vi "BMcalculate_v1_3 (slide_fix).vi"() -> ()   [LabVIEW 2014]
uses:
  <vilib>/Analysis/coordinate.llb/2D Cartesian Coordinate Rotation (Array).vi
  <vilib>/Analysis/baseanly.llb/Mean (DBL).vi
  <vilib>/Utility/file.llb/Read From Spreadsheet File (string).vi
  <vilib>/Utility/file.llb/Write To Spreadsheet File (DBL).vi
  <vilib>/Analysis/NI_AALBase.lvlib
  <vilib>/Analysis/NI_AALPro.lvlib
panel:
  in  "(T=X , F=Y)":bool=TRUE
  in  "Filter window size":i32=100
  out "Array":dbl[](array[numeric])
  out "created path 2":path
  out "created path":path
  in  "Save Time-trace":bool
  in  "nm/pixel":dbl=72.5 format="%#_13g"
  in  "Folder path":path
  in  "?":bool
  in  "~":dbl=1.15 format="%#_13g"
  in  "x/y for all":dbl=0.85 format="%#_13g"
  out "filename":string
  in  "Filter mode":T1(ring)=enum."Median_slide window"
  in  "Save to vertical data ?":bool
  in  "?":enum32{"slide by slide", "delay"}(tab)=enum."delay"
  in  "?":bool
  in  "seconds to wait":u32
  in  "?":dbl=7.963 format="%#_13g"
  in  "?":dbl=48.61 format="%#_13g"
  in  "Save BM":bool
  in  "?":bool=TRUE
  in  "Save X-Y plot":bool
  in  "less than":dbl=0.2 format="%#_13g"
  in  "?":bool
  in  "?":bool
  in  "?":bool=TRUE
  in  "?":T2(tab)
  out "Filenames":string[](array[string])
  out "useful AOIs":i32[](array[numeric])
  out "# of AOI":i32[](array[numeric])
  out "% of useful AOIs":dbl
  out "tt # of AOIs":i32
  out "# of Frames":dbl[](array[numeric])
  out "tt # 0f useful AOIs":i32
  out "?":T3(graph)
  out "size(s)":i32
  out "X-Y plot":cluster{dbl[], dbl[]}(graph)
  out "Xstd":dbl
  out "ystd":dbl[](array[numeric])
  out "X":dbl format="%0.2f"
  out "Y":dbl format="%0.2f"
  out "?":T3(graph)
  out "tt # of useful AOIs":i32
  out "xstd":dbl[](array[numeric])
  out "# of AOI":i32
  out "y 2":dbl[](array[numeric])
  out "# of frames":dbl
  out "all y position (pixel)":dbl[][](array[numeric])
  out "all x position (pixel)":dbl[][](array[numeric])
  out "y":dbl[](array[numeric])
  out "x":dbl[](array[numeric])
  out "y":dbl[](array[numeric])
  out "x":dbl[](array[numeric])
  out "number":dbl[][](array[numeric])
  out "all rows":string[][](array[string])
  out "Useful aoi number":string[][](array[string])
  in  "Tab Control":enum32{"Time trace"}(tab)
  out "Time trace":T4(graph)
  in  "Highlight":dbl=30.0
  in  "±":dbl=30.0
  out "aoi":string
  # "Critiria"
  # "±"
  # "nm"
  # "for ssDNA strande exchange \n                    23.776±6.613 nm"
  # "for D-loop  (90+4)\n                    48.61±7.963 nm"
  # "for D-loop  (150+4)\n                    49.57±8.56 nm"
  # "nm"
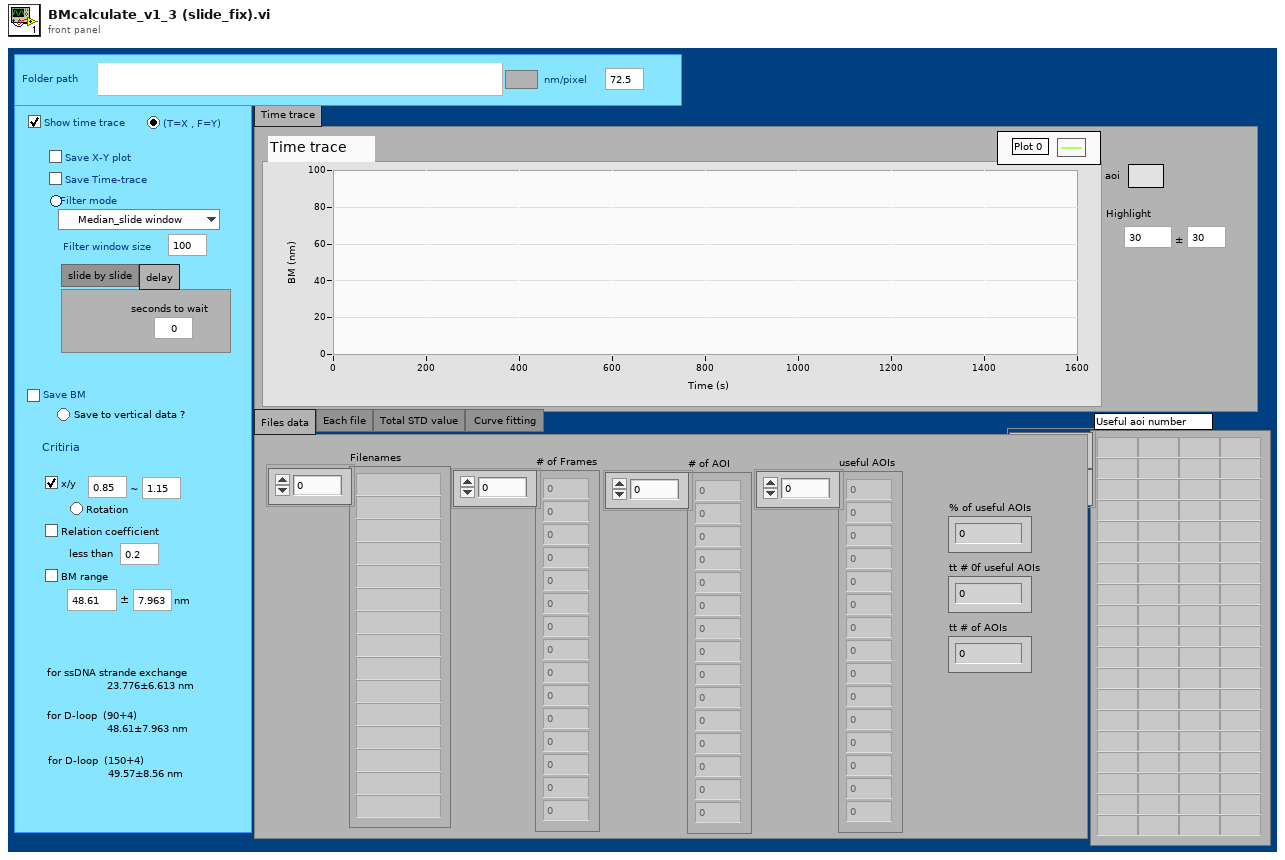
[diagram p1: front panel]
types:
  T1 = enum16{"Median_fix window", "Average_fix window", "Median_slide window", "Average_slide window"}
  T2 = enum32{"Files data", "Each file", "Total STD value", "Curve fitting "}
  T3 = cluster{"X Values":dbl[], "Histogram: h(x)":i32[]}
  T4 = cluster{"Filtered X":dbl[], "Filtered X":dbl[]}[]
  T5 = cluster{"all y position (pixel)":dbl[], "all x position (pixel)":dbl[]}
  T6 = cluster{"all x position (pixel)":dbl[], "all y position (pixel)":dbl[]}
  T7 = typedef "imagedata.ctl" = cluster{"image type":i32, "image depth":i32, "image":u8[], "mask":u8[], "colors":u32[], "Rectangle":cluster{"left":i16, "top":i16, "right":i16, "bottom":i16}}
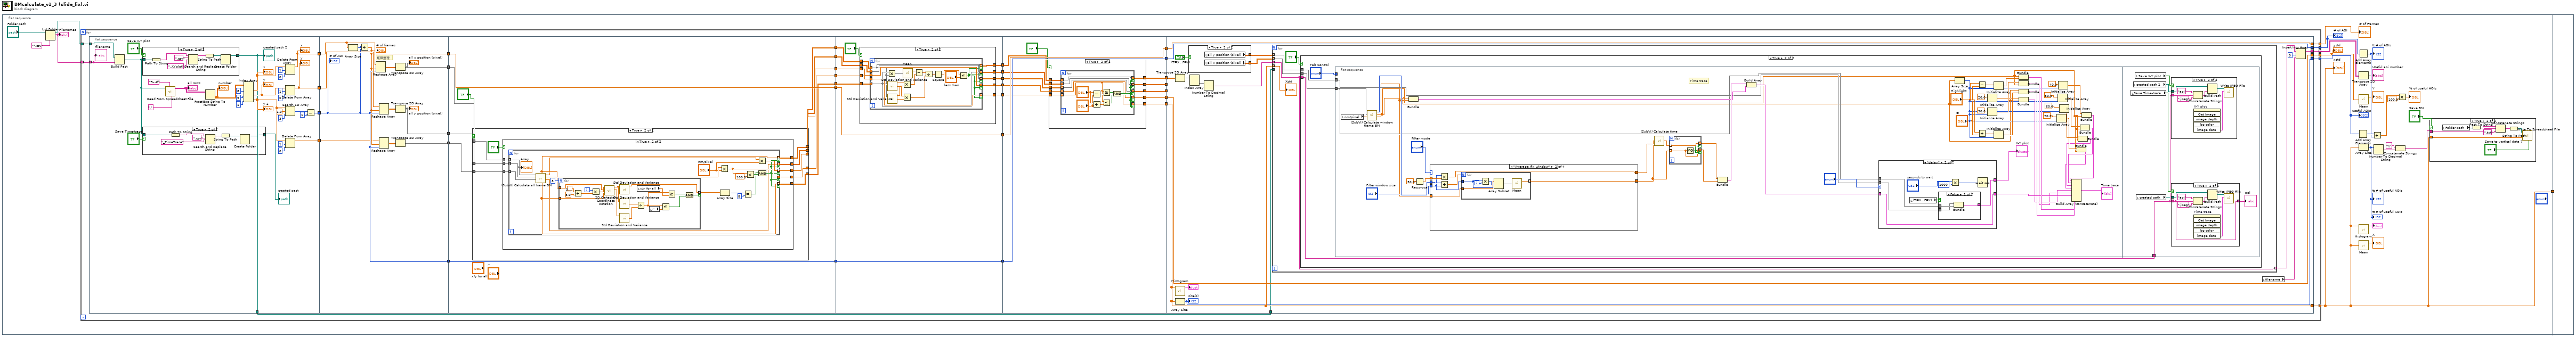
[diagram p0: block diagram]
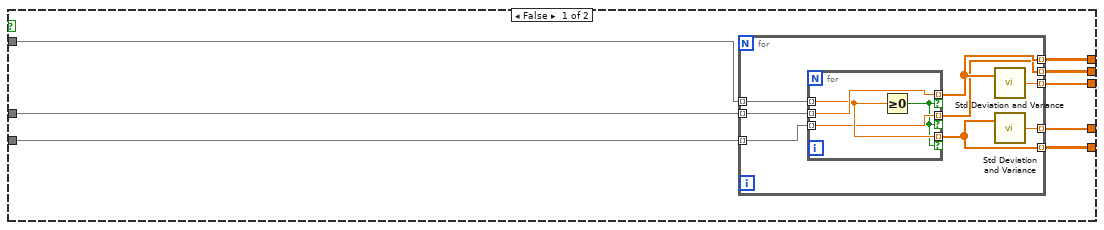
[diagram p5: hidden frame]
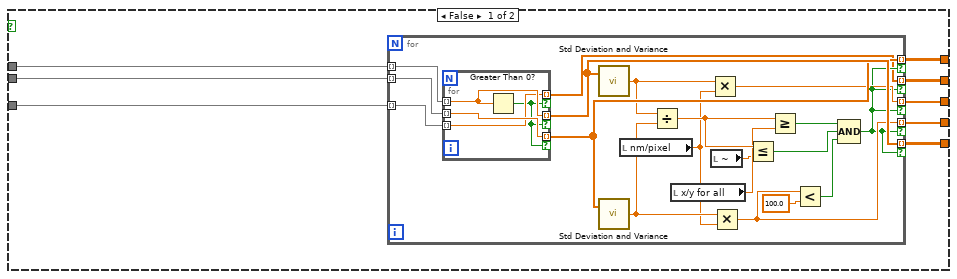
[diagram p6: hidden frame]
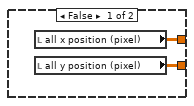
[diagram p9: hidden frame]
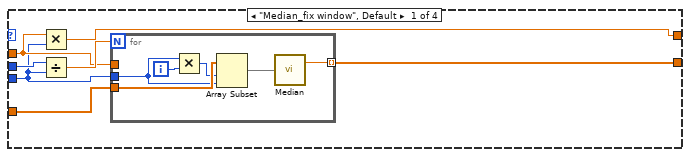
[diagram p11: hidden frame]
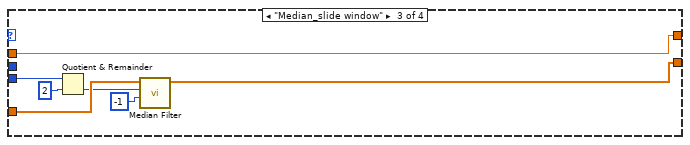
[diagram p12: hidden frame]
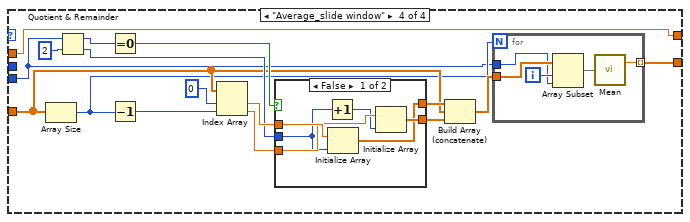
[diagram p13: hidden frame]
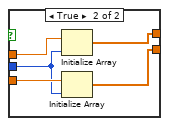
[diagram p14: hidden frame]
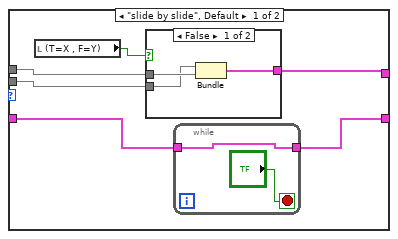
[diagram p15: hidden frame]
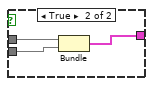
[diagram p16: hidden frame]
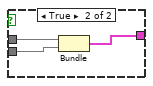
[diagram p17: hidden frame]
diagram:
  n1 = flat-sequence {
    tunnel: [w2] -> w1
    tunnel: w1 -> [_]
    frame #0 {
      n2 = List Folder(path="Folder path", pattern="*.csv") -> (path out=w24:path, filenames=w23:string[])  [unwired: 2 in, 2 out]
      "Filenames" <- w23
      n3 = for {
        tunnel: w24 -> [w37]
        tunnel: w23 -> [w72] mode=indexing
        tunnel: [w71] -> w2 mode=concatenating
        tunnel: [w70] -> w21 mode=indexing
        tunnel: [w69] -> w20 mode=indexing
        tunnel: [w68] -> w12 mode=concatenating
        tunnel: [w67] -> w13 mode=indexing
        tunnel: [w34] -> w4 mode=indexing
        n4 = flat-sequence {
          tunnel: [w92] -> w66
          tunnel: [w91] -> w65
          tunnel: [w85] -> w64
          tunnel: w37 -> [w80]
          tunnel: w72 -> [w76]
          tunnel: [w81] -> w41
          tunnel: [w79] -> w35
          tunnel: w66 -> [w128]
          tunnel: w65 -> [w127]
          tunnel: w64 -> [w126]
          tunnel: [w125] -> w63
          tunnel: [w126] -> w62
          tunnel: [w121] -> w61
          tunnel: [w120] -> w60
          tunnel: w41 -> [w124]
          tunnel: [w122] -> w40
          tunnel: w63 -> [w142]
          tunnel: w62 -> [w141]
          tunnel: w61 -> [w140]
          tunnel: w60 -> [w139]
          tunnel: [w141] -> w53
          tunnel: [w142] -> w51
          tunnel: [w137] -> w49
          tunnel: [w136] -> w47
          tunnel: [w135] -> w45
          tunnel: [w134] -> w43
          tunnel: w40 -> [w132]
          tunnel: [w133] -> w39
          tunnel: w53 -> [w260]
          tunnel: [w260] -> w52
          tunnel: w51 -> [w259]
          tunnel: [w259] -> w50
          tunnel: w49 -> [w255]
          tunnel: [w250] -> w48
          tunnel: w47 -> [w258]
          tunnel: [w253] -> w46
          tunnel: w45 -> [w257]
          tunnel: [w252] -> w44
          tunnel: w43 -> [w256]
          tunnel: [w251] -> w42
          tunnel: w39 -> [w249]
          tunnel: [w248] -> w38
          tunnel: w52 -> [w306]
          tunnel: w50 -> [w305]
          tunnel: w48 -> [w300]
          tunnel: [w306] -> w59
          tunnel: [w305] -> w58
          tunnel: [w299] -> w57
          tunnel: [w303] -> w56
          tunnel: w46 -> [w304]
          tunnel: [w301] -> w55
          tunnel: w44 -> [w302]
          tunnel: [w294] -> w54
          tunnel: w42 -> [w295]
          tunnel: w38 -> [w297]
          tunnel: [w296] -> w36
          tunnel: [w351] -> w68
          tunnel: [w352] -> w67
          tunnel: [w353] -> w69
          tunnel: [w349] -> w70
          tunnel: [w343] -> w71
          tunnel: w59 -> [w353]
          tunnel: w58 -> [w352]
          tunnel: w57 -> [w351]
          tunnel: w56 -> [_]
          tunnel: w55 -> [_]
          tunnel: w54 -> [w343]
          tunnel: w36 -> [w348]
          tunnel: w35 -> [w344]
          tunnel: [w339] -> w34
          frame #0 {
            n5 = Build Path(base path=w80, name or relative path=w76) -> (appended path=w74:path)
            n6 = case shown="True" "Save X-Y plot" {
              tunnel: w74 -> [w112 w119]
              tunnel: [w112 w113] -> w79
              frame False {
              }
              frame True {
                n7 = Path To String(path=w119) -> (string=w118:string)
                n8 = Search and Replace String(input string=w118, search string=".csv", replace string="_XYplot" ("replace string (\"\")")) -> (result string=w115:string)  [unwired: 5 in, 3 out]
                n9 = String To Path(string=w115) -> (path=w114:path)
                n10 = Create Folder(path (use dialog)=w114) -> (created path=w113:path)  [unwired: 2 in, 2 out]
              }
            }
            "created path 2" <- w79
            n11 = case shown="True" "Save Time-trace" {
              tunnel: w74 -> [w104 w111]
              tunnel: [w104 w105] -> w73
              frame False {
              }
              frame True {
                n12 = Path To String(path=w111) -> (string=w110:string)
                n13 = Search and Replace String(input string=w110, search string=".csv", replace string="_TimeTrace" ("replace string (\"\")")) -> (result string=w107:string)  [unwired: 5 in, 3 out]
                n14 = String To Path(string=w107) -> (path=w106:path)
                n15 = Create Folder(path (use dialog)=w106) -> (created path=w105:path)  [unwired: 2 in, 2 out]
              }
            }
            "created path" <- w73
            n16 = call-poly <vilib>:"Read From Spreadsheet File.vi"("delimiter (\\t)"="," ("delimiter (\\t)"), "format (%s)"="%.4f" ("format (%.3f)"), "file path (dialog if empty)"=w74) -> ("all rows"=w102:string[][])  [unwired: 4 in, 4 out]
            "all rows" <- w102
            n17 = Fract/Exp String To Number(string=w102) -> (number=w101:dbl[][])  [unwired: 3 in, 1 out]
            "number" <- w101
            n18 = Index Array(array=w101, index (col) #1=8 ("disabled index (col)"), index (col) #2=9 ("index (col)"), index (col) #3=1 ("index (col)")) -> (element #1=w93:dbl[], element #2=w94:dbl[], element #3=w82:dbl[])  [unwired: 3 in]
            "x" <- w93
            "y" <- w94
            "y 2" <- w82
            n19 = Delete From Array(array=w93, length=1, index=0) -> (array with subset deleted=w92:dbl[])  [unwired: 1 out]
            "x" <- w92
            n20 = Delete From Array(array=w94, length=1, index=0) -> (array with subset deleted=w91:dbl[])  [unwired: 1 out]
            "y" <- w91
            n21 = Search 1D Array(1D array=w82, element=1.0, start index (0)=3) -> (index of element=w87:i32)
            n22 = Delete From Array(array=w82, length=1, index=0) -> (array with subset deleted=w81:dbl[])  [unwired: 1 out]
            n23 = Subtract(x=w87, y=1) -> (x-y=w85:i32)
            "filename" <- w76
          }
          frame #1 {
            # "矩陣整理"
            n24 = Array Size(array=w128) -> (size(s)=w129:i32)
            n25 = Divide(x=w129, y=w126) -> (x/y=w125:dbl)
            "# of frames" <- w125
            n26 = Reshape Array(w128, w125, w126) -> (w130:dbl[][])
            n27 = Reshape Array(w127, w125, w126) -> (w131:dbl[][])
            n28 = Reshape Array(w124, w125, w126) -> (w123:dbl[][])
            n29 = Transpose 2D Array(2D array=w130) -> (transposed array=w121:dbl[][])
            "all x position (pixel)" <- w121
            n30 = Transpose 2D Array(2D array=w131) -> (transposed array=w120:dbl[][])
            "all y position (pixel)" <- w120
            n31 = Transpose 2D Array(2D array=w123) -> (transposed array=w122:dbl[][])
            "# of AOI" <- w126
          }
          frame #2 {
            n32 = case shown="True" "?" {
              tunnel: [w148 w171] -> w136
              tunnel: [w147 w170] -> w135
              tunnel: w140 -> [w150 w169]
              tunnel: w139 -> [w149 w168]
              tunnel: [w146 w167] -> w134
              tunnel: [w145 w166] -> w137
              tunnel: w132 -> [w144 w164]
              tunnel: [w143 w163] -> w133
              frame False {
                n33 = for {
                  tunnel: w150 -> [w158] mode=indexing
                  tunnel: w149 -> [w157] mode=indexing
                  tunnel: [w156] -> w148 mode=indexing
                  tunnel: [w155] -> w147 mode=indexing
                  tunnel: [w154] -> w146 mode=indexing
                  tunnel: [w153] -> w145 mode=indexing
                  tunnel: w144 -> [w152] mode=indexing
                  tunnel: [w151] -> w143 mode=indexing
                  n34 = for {
                    tunnel: w158 -> [w161] mode=indexing
                    tunnel: w157 -> [w162] mode=indexing
                    tunnel: [w161] -> w156 mode=indexing if=w159
                    tunnel: [w162] -> w155 mode=indexing if=w159
                    tunnel: w152 -> [w160] mode=indexing
                    tunnel: [w160] -> w151 mode=indexing if=w159
                    n35 = Greater Or Equal To 0?(x=w161) -> (x >= 0?=w159:bool)
                  }
                  n36 = call <vilib>:"Std Deviation and Variance.vi"("X"=w155) -> ("standard deviation"=w153:dbl)  [unwired: 1 in, 2 out]
                  n37 = call <vilib>:"Std Deviation and Variance.vi"("X"=w156) -> ("standard deviation"=w154:dbl)  [unwired: 1 in, 2 out]
                }
              }
              frame True {
                n38 = case shown="True" "?" {
                  tunnel: w168 -> [w178 w210]
                  tunnel: w169 -> [w179 w209]
                  tunnel: [w177 w208] -> w171
                  tunnel: [w176 w207] -> w170
                  tunnel: [w175 w206] -> w167
                  tunnel: [w174 w205] -> w166
                  tunnel: w164 -> [w173 w204]
                  tunnel: [w172 w203] -> w163
                  frame False {
                    n39 = for {
                      tunnel: w179 -> [w198] mode=indexing
                      tunnel: w178 -> [w197] mode=indexing
                      tunnel: [w196] -> w177 mode=indexing if=w183
                      tunnel: [w195] -> w176 mode=indexing if=w183
                      tunnel: [w184] -> w175 mode=indexing if=w183
                      tunnel: [w187] -> w174 mode=indexing if=w183
                      tunnel: [w181] -> w172 mode=indexing if=w183
                      tunnel: w173 -> [w182] mode=indexing
                      n40 = for {
                        tunnel: w198 -> [w201] mode=indexing
                        tunnel: w197 -> [w202] mode=indexing
                        tunnel: [w201] -> w196 mode=indexing if=w199
                        tunnel: [w202] -> w195 mode=indexing if=w199
                        tunnel: w182 -> [w200] mode=indexing
                        tunnel: [w200] -> w181 mode=indexing if=w199
                        n41 = Greater Than 0?(x=w201) -> (x > 0?=w199:bool)
                      }
                      n42 = call <vilib>:"Std Deviation and Variance.vi"("X"=w196) -> ("standard deviation"=w188:dbl)  [unwired: 1 in, 2 out]
                      n43 = call <vilib>:"Std Deviation and Variance.vi"("X"=w195) -> ("standard deviation"=w189:dbl)  [unwired: 1 in, 2 out]
                      n44 = local read "nm/pixel"() -> (w180:dbl)
                      n45 = Divide(x=w188, y=w189) -> (x/y=w194:dbl)
                      n46 = local read "x/y for all"() -> (w193:dbl)
                      n47 = Multiply(x=w188, y=w180) -> (x*y=w187:dbl)
                      n48 = local read "~"() -> (w192:dbl)
                      n49 = Multiply(x=w189, y=w180) -> (x*y=w184:dbl)
                      n50 = Less Or Equal?(x=w194, y=w192) -> (x <= y?=w190:bool)
                      n51 = Greater Or Equal?(x=w194, y=w193) -> (x >= y?=w191:bool)
                      n52 = Less?(x=w184, y=100.0) -> (x < y?=w185:bool)
                      n53 = Compound Arithmetic op=AND(w191, w190, w185) -> (w183:bool)
                    }
                  }
                  frame True {
                    n54 = for {
                      tunnel: w209 -> [w229] mode=indexing
                      tunnel: w210 -> [w228] mode=indexing
                      tunnel: [w214] -> w206 mode=indexing if=w213
                      tunnel: [w221] -> w207 mode=indexing if=w213
                      tunnel: [w222] -> w208 mode=indexing if=w213
                      tunnel: [w219] -> w205 mode=indexing if=w213
                      tunnel: [w212] -> w203 mode=indexing if=w213
                      tunnel: w204 -> [w211] mode=indexing
                      n55 = call "(SubVI) Calculate all frame BM.vi"("AOI label"=w211, "y position (pixel)"=w228, "x position (pixel)"=w229) -> ("Array out"=w212:dbl[], "standard deviation 2"=w223:dbl, "standard deviation"=w220:dbl, "Array 4"=w222:dbl[], "Array 3"=w221:dbl[])  [unwired: 4 in]
                      n56 = for {
                        N: 8 -> [_]
                        tunnel: w222 -> [w242]
                        tunnel: w221 -> [w241]
                        tunnel: [w233] -> w224 mode=indexing if=w232
                        i -> [w243]
                        n57 = Divide(x=3.141592653589793, y=8.0) -> (x/y=w246:dbl)
                        n58 = Multiply(x=w243, y=w246) -> (x*y=w244:dbl)
                        n59 = call-poly <vilib>:"2D Cartesian Coordinate Rotation.vi"("theta"=w244, "Y"=w241, "X"=w242) -> ("Y Out"=w234:dbl[], "X Out"=w235:dbl[])  [unwired: 6 in, 1 out]
                        n60 = call <vilib>:"Std Deviation and Variance.vi"("X"=w235) -> ("mean"=w233:dbl)  [unwired: 1 in, 2 out]
                        n61 = call <vilib>:"Std Deviation and Variance.vi"("X"=w235) -> ("standard deviation"=w240:dbl)  [unwired: 1 in, 2 out]
                        n62 = call <vilib>:"Std Deviation and Variance.vi"("X"=w234) -> ("standard deviation"=w239:dbl)  [unwired: 1 in, 2 out]
                        n63 = Divide(x=w240, y=w239) -> (x/y=w238:dbl)
                        n64 = local read "x/y for all"() -> (w231:dbl)
                        n65 = local read "~"() -> (w230:dbl)
                        n66 = Less Or Equal?(x=w238, y=w230) -> (x <= y?=w236:bool)
                        n67 = Greater Or Equal?(x=w238, y=w231) -> (x >= y?=w237:bool)
                        n68 = Compound Arithmetic op=AND(w237, w236) -> (w232:bool)
                      }
                      n69 = Multiply(x=w223, y="nm/pixel") -> (x*y=w214:dbl)
                      n70 = Array Size(array=w224) -> (size(s)=w226:i32)
                      n71 = Equal?(x=w226, y=8) -> (x = y?=w215:bool)
                      n72 = Less?(x=w214, y=100.0) -> (x < y?=w216:bool)
                      n73 = Multiply(x=w220, y="nm/pixel") -> (x*y=w219:dbl)
                      n74 = Compound Arithmetic op=AND(w215, w216) -> (w213:bool)
                      "Array" <- w229
                    }
                  }
                }
              }
            }
          }
          frame #3 {
            n75 = case shown="True" "?" {
              tunnel: w258 -> [w265 w275]
              tunnel: w257 -> [w264 w274]
              tunnel: w256 -> [w263 w271]
              tunnel: w255 -> [w262 w269]
              tunnel: [w265 w273] -> w253
              tunnel: [w264 w272] -> w252
              tunnel: [w263 w270] -> w251
              tunnel: [w262 w268] -> w250
              tunnel: w249 -> [w261 w267]
              tunnel: [w261 w266] -> w248
              frame False {
              }
              frame True {
                n76 = for {
                  tunnel: w275 -> [w281] mode=indexing
                  tunnel: w274 -> [w280] mode=indexing
                  tunnel: [w281] -> w273 mode=indexing if=w276
                  tunnel: [w280] -> w272 mode=indexing if=w276
                  tunnel: [w288] -> w270 mode=indexing if=w276
                  tunnel: w271 -> [w288] mode=indexing
                  tunnel: w269 -> [w287] mode=indexing
                  tunnel: [w287] -> w268 mode=indexing if=w276
                  tunnel: [w277] -> w266 mode=indexing if=w276
                  tunnel: w267 -> [w277] mode=indexing
                  n77 = Multiply(x=w281, y=w280) -> (x*y=w279:dbl[])
                  n78 = call <vilib>:"Std Deviation and Variance.vi"("X"=w281) -> ("mean"=w284:dbl, "standard deviation"=w286:dbl)  [unwired: 1 in, 1 out]
                  n79 = call <vilib>:"Std Deviation and Variance.vi"("X"=w280) -> ("mean"=w283:dbl, "standard deviation"=w285:dbl)  [unwired: 1 in, 1 out]
                  n80 = Multiply(x=w284, y=w283) -> (x*y=w282:dbl)
                  n81 = Multiply(x=w286, y=w285) -> (x*y=w289:dbl)
                  n82 = call-poly <vilib>:"Mean.vi"("X"=w279) -> ("mean"=w278:dbl)  [unwired: 1 out]
                  n83 = Subtract(x=w278, y=w282) -> (x-y=w290:dbl)
                  n84 = Divide(x=w290, y=w289) -> (x/y=w291:dbl)
                  n85 = Square(x=w291) -> (x^2=w292:dbl)
                  n86 = Less Or Equal?(x=w292, y="less than") -> (x <= y?=w276:bool)
                }
              }
            }
          }
          frame #4 {
            n87 = case shown="True" "?" {
              tunnel: [w312 w322] -> w303
              tunnel: w304 -> [w312 w323]
              tunnel: w302 -> [w311 w321]
              tunnel: [w311 w320] -> w301
              tunnel: w295 -> [w310 w319]
              tunnel: [w310 w318] -> w294
              tunnel: w300 -> [w309 w317]
              tunnel: [w309 w316] -> w299
              tunnel: w297 -> [w308 w315]
              tunnel: [w307 w314] -> w296
              frame False {
                n88 = for {
                  tunnel: w308 -> [w313] mode=indexing
                  tunnel: [w313] -> w307 mode=indexing
                }
              }
              frame True {
                n89 = for {
                  tunnel: [w335] -> w322 mode=indexing if=w330
                  tunnel: w323 -> [w335] mode=indexing
                  tunnel: [w334] -> w320 mode=indexing if=w330
                  tunnel: w321 -> [w334] mode=indexing
                  tunnel: [w324] -> w318 mode=indexing if=w330
                  tunnel: w319 -> [w324] mode=indexing
                  tunnel: w317 -> [w329] mode=indexing
                  tunnel: [w329] -> w316 mode=indexing if=w330
                  tunnel: [w331] -> w314 mode=indexing if=w330
                  tunnel: w315 -> [w331] mode=indexing
                  n90 = Subtract(x="?", y="?") -> (x-y=w326:dbl)
                  n91 = Add(x="?", y="?") -> (x+y=w325:dbl)
                  n92 = Greater Or Equal?(x=w324, y=w326) -> (x >= y?=w333:bool)
                  n93 = Less Or Equal?(x=w324, y=w325) -> (x <= y?=w332:bool)
                  n94 = Compound Arithmetic op=AND(w333, w332) -> (w330:bool)
                }
              }
            }
          }
          frame #5 {
            n95 = Transpose 2D Array(2D array=w348) -> (transposed array=w347:dbl[][])
            n96 = call <vilib>:"Histogram.vi"("X"=w343) -> ("Histogram Graph"=→"?":T3)  [unwired: 7 in, 3 out]
            n97 = Array Size(array=w343) -> (size(s)=w349:i32)
            "size(s)" <- w349
            n98 = case shown="True" "(T=X , F=Y)" {
              tunnel: [w355 w357] -> w337
              tunnel: [w354 w356] -> w336
              frame False {
                n99 = local read "all x position (pixel)"() -> (w354:dbl[][])
                n100 = local read "all y position (pixel)"() -> (w355:dbl[][])
              }
              frame True {
                n101 = local read "all y position (pixel)"() -> (w356:dbl[][])
                n102 = local read "all x position (pixel)"() -> (w357:dbl[][])
              }
            }
            n103 = Index Array(array=w347) -> (element=w346:dbl[])  [unwired: 2 in]
            n104 = Number To Decimal String(number=w346) -> (decimal integer string=w345:string[])  [unwired: 1 in]
            n105 = for {
              tunnel: w337 -> [w361] mode=indexing
              tunnel: w336 -> [w362] mode=indexing
              tunnel: w345 -> [w358] mode=indexing
              tunnel: w344 -> [_]
              tunnel: w343 -> [w359] mode=indexing
              tunnel: [w358] -> w340 mode=indexing
              n106 = case shown="True" "?" {
                tunnel: w362 -> [_ w366]
                tunnel: w361 -> [_ w365]
                tunnel: w358 -> [_ w364]
                frame False {
                }
                frame True {
                  n107 = flat-sequence {
                    tunnel: w366 -> [w406]
                    tunnel: w365 -> [w405]
                    tunnel: "Tab Control" -> [_]
                    tunnel: w364 -> [w516]
                    frame #0 {
                      # "Time trace"
                      n108 = local read "nm/pixel"() -> (w393:dbl)
                      n109 = call "(SubVI) Calculate window frame BM.vi"("nm/pixel"=w393, "all x position (pixel)"=w405) -> ("BM"=w388:dbl[], "sec"=w371:dbl[], "frame"=w411:i32)  [unwired: 3 in]
                      n110 = Bundle("sec"=w371, "BM"=w388) -> (w410:cluster{"sec":dbl[], "BM":dbl[]})  [unwired: 1 in]
                      n111 = Reciprocal(x=30.0) -> (1/x=w390:dbl)
                      n112 = case shown="\"Average_fix window\"" "Filter mode" {
                        tunnel: [w424 w435 w450 w467] -> w387
                        tunnel: w388 -> [w425 w436 w451 w456]
                        tunnel: w411 -> [w423 w438 _ _]
                        tunnel: "Filter window size" -> [w419 w432 w447 w453]
                        tunnel: w390 -> [w421 w434 w449 w452]
                        tunnel: [w420 w433 w449 w452] -> w389
                        frame "Median_fix window", Default {
                          n113 = Multiply(x=w421, y=w419) -> (x*y=w420:dbl)
                          n114 = Divide(x=w423, y=w419) -> (x/y=w422:dbl)
                          n115 = for {
                            N: w422 -> [_]
                            tunnel: w425 -> [w431]
                            tunnel: [w429] -> w424 mode=indexing
                            tunnel: w419 -> [w426]
                            tunnel: w421 -> [_]
                            i -> [w428]
                            n116 = Multiply(x=w426, y=w428) -> (x*y=w427:i32)
                            n117 = Array Subset(array=w431, index=w427, length=w426) -> (w430:dbl[])
                            n118 = call <vilib>:"Median.vi"("X"=w430) -> ("median"=w429:dbl)  [unwired: 1 out]
                          }
                        }
                        frame "Average_fix window" {
                          n119 = Multiply(x=w432, y=w434) -> (x*y=w433:dbl)
                          n120 = Divide(x=w438, y=w432) -> (x/y=w437:dbl)
                          n121 = for {
                            N: w437 -> [_]
                            tunnel: w436 -> [w444]
                            tunnel: [w442] -> w435 mode=indexing
                            tunnel: w432 -> [w440]
                            i -> [w441]
                            n122 = Multiply(x=w440, y=w441) -> (x*y=w439:i32)
                            n123 = Array Subset(array=w444, index=w439, length=w440) -> (w443:dbl[])
                            n124 = call-poly <vilib>:"Mean.vi"("X"=w443) -> ("mean"=w442:dbl)  [unwired: 1 out]
                          }
                        }
                        frame "Median_slide window" {
                          n125 = Quotient & Remainder(x=w447, y=2) -> (floor(x/y)=w445:i32)  [unwired: 1 out]
                          n126 = call <vilib>:"Median Filter.vi"("right rank"=-1, "left rank"=w445, "X"=w451) -> ("Filtered X"=w450:dbl[])  [unwired: 7 in, 1 out]
                        }
                        frame "Average_slide window" {
                          n127 = Array Size(array=w456) -> (size(s)=w454:i32)
                          n128 = Quotient & Remainder(x=w453, y=2) -> (x-y*floor(x/y)=w463:i32, floor(x/y)=w461:i32)
                          n129 = Equal To 0?(x=w463) -> (x = 0?=w462:bool)
                          n130 = Decrement(x=w454) -> (x-1=w460:i32)
                          n131 = Index Array(array=w456, index #1=0 ("index"), index #2=w460) -> (element #1=w465:dbl, element #2=w459:dbl)
                          n132 = case shown="False" w462 {
                            tunnel: w465 -> [w473 w478]
                            tunnel: w461 -> [w470 w476]
                            tunnel: w459 -> [w472 w477]
                            tunnel: [w468 w475] -> w458
                            tunnel: [w469 w474] -> w457
                            frame False {
                              n133 = Increment(x=w470) -> (x+1=w471:i32)
                              n134 = Initialize Array(w473, w470) -> (w468:dbl[])
                              n135 = Initialize Array(w472, w471) -> (w469:dbl[])
                            }
                            frame True {
                              n136 = Initialize Array(w478, w476) -> (w475:dbl[])
                              n137 = Initialize Array(w477, w476) -> (w474:dbl[])
                            }
                          }
                          n138 = Build Array (concatenate)(w458, w456, w457) -> (w455:dbl[])
                          n139 = for {
                            N: w454 -> [_]
                            tunnel: w455 -> [w483]
                            tunnel: [w481] -> w467 mode=indexing
                            tunnel: w453 -> [w479]
                            i -> [w480]
                            n140 = Array Subset(array=w483, index=w480, length=w479) -> (w482:dbl[])
                            n141 = call-poly <vilib>:"Mean.vi"("X"=w482) -> ("mean"=w481:dbl)  [unwired: 1 out]
                          }
                        }
                      }
                      n142 = call "(SubVI) Calculate time.vi"("dt"=w389, "BM"=w387) -> ("Time (s)"=w386:dbl[])  [unwired: 3 in]
                      n143 = for {
                        tunnel: w387 -> [w416] mode=indexing
                        tunnel: [w416] -> w384 mode=indexing if=w417
                        tunnel: w386 -> [w418] mode=indexing
                        tunnel: [w418] -> w385 mode=indexing if=w417
                        n144 = Not Equal To 0?(x=w416) -> (x != 0?=w417:bool)
                      }
                      n145 = Bundle(w385, w384) -> (w415:cluster{dbl[], dbl[]})  [unwired: 1 in]
                      n146 = Build Array(w415, w410) -> (w414:cluster{"sec":dbl[], "BM":dbl[]}[])
                      n147 = case shown="\"delay\"" "?" {
                        tunnel: w414 -> [w489 w505]
                        tunnel: [w488 w505] -> w407
                        tunnel: w405 -> [w487 w501]
                        tunnel: w406 -> [w486 w500]
                        tunnel: [w485 w499] -> w409
                        frame "slide by slide", Default {
                          n148 = local read "(T=X , F=Y)"() -> (w484:bool)
                          n149 = case shown="False" w484 {
                            tunnel: w487 -> [w492 w495]
                            tunnel: w486 -> [w491 w494]
                            tunnel: [w490 w493] -> w485
                            frame False {
                              n150 = Bundle("all y position (pixel)"=w491, "all x position (pixel)"=w492) -> (w490:T5)  [unwired: 1 in]
                            }
                            frame True {
                              n151 = Bundle("all x position (pixel)"=w495, "all y position (pixel)"=w494) -> (w493:T6)  [unwired: 1 in]
                            }
                          }
                          n152 = while {
                            tunnel: w489 -> [w496]
                            tunnel: [w496] -> w488
                            stop <- "?" stop-if-true
                          }
                        }
                        frame "delay" {
                          n153 = local read "(T=X , F=Y)"() -> (w498:bool)
                          n154 = case shown="False" w498 {
                            tunnel: w501 -> [w508 w511]
                            tunnel: w500 -> [w507 w510]
                            tunnel: [w506 w509] -> w499
                            frame False {
                              n155 = Bundle("all y position (pixel)"=w507, "all x position (pixel)"=w508) -> (w506:T5)  [unwired: 1 in]
                            }
                            frame True {
                              n156 = Bundle("all x position (pixel)"=w511, "all y position (pixel)"=w510) -> (w509:T6)  [unwired: 1 in]
                            }
                          }
                          n157 = Multiply(x="seconds to wait", y=u32 1000) -> (x*y=w503:u32)
                          n158 = Wait (ms)(milliseconds to wait=w503) -> ()  [unwired: 1 out]
                        }
                      }
                      "X-Y plot" <- w409
                      n159 = Array Size(array=w371) -> (size(s)=w377:i32)
                      n160 = Subtract(x="Highlight", y="±") -> (x-y=w399:dbl)
                      n161 = Add(x="Highlight", y="±") -> (x+y=w398:dbl)
                      n162 = Initialize Array(20.0 ("element"), w377) -> (w397:dbl[])
                      n163 = Initialize Array(30.0 ("element"), w377) -> (w394:dbl[])
                      n164 = Initialize Array(w399, w377) -> (w404:dbl[])
                      n165 = Initialize Array(w398, w377) -> (w403:dbl[])
                      n166 = Bundle("sec"=w371, w404) -> (w408:cluster{"sec":dbl[], dbl[]})  [unwired: 1 in]
                      n167 = Bundle(w394, "sec"=w371) -> (w382:cluster{dbl[], "sec":dbl[]})  [unwired: 1 in]
                      n168 = Bundle("sec"=w371, w403) -> (w402:cluster{"sec":dbl[], dbl[]})  [unwired: 1 in]
                      n169 = Bundle(w397, "sec"=w371) -> (w383:cluster{dbl[], "sec":dbl[]})  [unwired: 1 in]
                      n170 = Initialize Array(70.0 ("element"), w377) -> (w372:dbl[])
                      n171 = Initialize Array(50.0 ("element"), w377) -> (w374:dbl[])
                      n172 = Initialize Array(40.0 ("element"), w377) -> (w375:dbl[])
                      n173 = Initialize Array(60.0 ("element"), w377) -> (w373:dbl[])
                      n174 = Bundle(w372, "sec"=w371) -> (w367:cluster{dbl[], "sec":dbl[]})  [unwired: 1 in]
                      n175 = Bundle(w373, "sec"=w371) -> (w368:cluster{dbl[], "sec":dbl[]})  [unwired: 1 in]
                      n176 = Bundle(w374, "sec"=w371) -> (w369:cluster{dbl[], "sec":dbl[]})  [unwired: 1 in]
                      n177 = Bundle(w375, "sec"=w371) -> (w370:cluster{dbl[], "sec":dbl[]})  [unwired: 1 in]
                      n178 = Build Array (concatenate)(w370, w369, w368, w367, w383, w382, w407, w408, w402) -> (→"Time trace":cluster{"sec":dbl[], "BM":dbl[]}[])
                    }
                    frame #1 {
                      n179 = local read "Save Time-trace"() -> (w517:bool)
                      n180 = local read "created path 2"() -> (w513:path)
                      n181 = local read "Save X-Y plot"() -> (w514:bool)
                      n182 = local read "created path"() -> (w515:path)
                      n183 = case shown="True" w514 {
                        tunnel: w516 -> [_ w524]
                        tunnel: w513 -> [_ w521]
                        frame False {
                        }
                        frame True {
                          n184 = Concatenate Strings("aoi" ("string"), w524, ".jpeg" ("string")) -> (w522:string)
                          n185 = invoke on="X-Y plot" class="XYGraph (strict)" method="Get Image"() -> ("image data"=w519:T7)  [unwired: 6 in, 5 out]
                          n186 = Build Path(base path=w521, name or relative path=w522) -> (appended path=w520:path)
                          n187 = call <vilib>:"Write JPEG File.vi"("image data"=w519, "path to JPEG file"=w520) -> ()  [unwired: 8 in, 2 out]
                        }
                      }
                      n188 = case shown="True" w517 {
                        tunnel: w516 -> [w525 w527]
                        tunnel: w515 -> [_ w530]
                        tunnel: [w525 w527] -> w512
                        frame False {
                        }
                        frame True {
                          n189 = Concatenate Strings("aoi" ("string"), w527, ".jpeg" ("string")) -> (w531:string)
                          n190 = invoke on="Time trace" class="XYGraph (strict)" method="Get Image"() -> ("image data"=w526:T7)  [unwired: 6 in, 5 out]
                          n191 = Build Path(base path=w530, name or relative path=w531) -> (appended path=w529:path)
                          n192 = call <vilib>:"Write JPEG File.vi"("image data"=w526, "path to JPEG file"=w529) -> ()  [unwired: 8 in, 2 out]
                        }
                      }
                      "aoi" <- w512
                    }
                  }
                }
              }
              "Xstd" <- w359
            }
            n193 = local read "filename"() -> (w342:string)
            n194 = Insert Into Array(array=w340, index=0, new element=w342) -> (w339:string[])
          }
        }
      }
      "useful AOIs" <- w21
      "# of AOI" <- w20
      "ystd" <- w12
      "# of Frames" <- w13
      "xstd" <- w2
      n195 = Add Array Elements(numeric array=w21) -> (sum=w19:i32)
      n196 = Add Array Elements(numeric array=w20) -> (sum=w18:i32)
      "tt # of AOIs" <- w18
      n197 = Transpose 2D Array(2D array=w4) -> (transposed array=→"Useful aoi number":string[][])
      n198 = call-poly <vilib>:"Mean.vi"("X"=w12) -> ("mean"=→"Y":dbl)  [unwired: 1 out]
      n199 = Array Size(array=w2) -> (size(s)=w9:i32)
      "tt # 0f useful AOIs" <- w9
      "tt # of useful AOIs" <- w9
      n200 = call <vilib>:"Histogram.vi"("X"=w2) -> ("Histogram Graph"=→"?":T3)  [unwired: 7 in, 3 out]
      n201 = call-poly <vilib>:"Mean.vi"("X"=w2) -> ("mean"=→"X":dbl)  [unwired: 1 out]
      n202 = Divide(x=w19, y=w18) -> (x/y=w17:dbl)
      n203 = Number To Decimal String(number=w9) -> (decimal integer string=w7:string)  [unwired: 1 in]
      n204 = Concatenate Strings("\\" ("string"), w7) -> (w6:string)
      n205 = Multiply(x=w17, y=100.0) -> (x*y=→"% of useful AOIs":dbl)
      n206 = case shown="True" "Save BM" {
        tunnel: w2 -> [_ w33]
        tunnel: w6 -> [_ w27]
        frame False {
        }
        frame True {
          n207 = local read "Folder path"() -> (w32:path)
          n208 = Path To String(path=w32) -> (string=w31:string)
          n209 = Concatenate Strings(w31, w27, ".txt" ("string")) -> (w30:string)
          n210 = String To Path(string=w30) -> (path=w29:path)
          n211 = call-poly <vilib>:"Write To Spreadsheet File.vi"("transpose? (no:F)"="Save to vertical data ?", "1D data"=w33, "file path (dialog if empty)"=w29) -> ()  [unwired: 5 in, 1 out]
        }
      }
    }
    frame #1 {
    }
  }
